vi "Set Photon Counting Threshold.vi"(8 "error in (no error)":errorcluster, 10 "max":i32, 11 "min":i32) -> (0 "error out":errorcluster, 3 "function return":u32)   [LabVIEW 2014, in "atmcd32d.lvlib"]
doc: "unsigned int WINAPI SetPhotonCountingThreshold(long min, long max);"
uses:
  atmcd32d.lvlib
  atmcd32d.dll
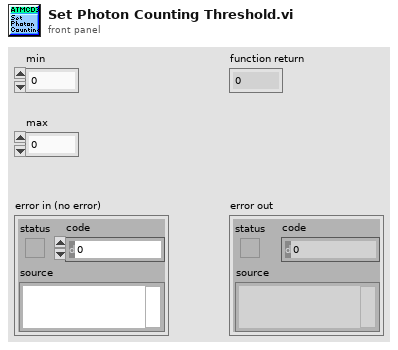
[diagram p1: front panel]
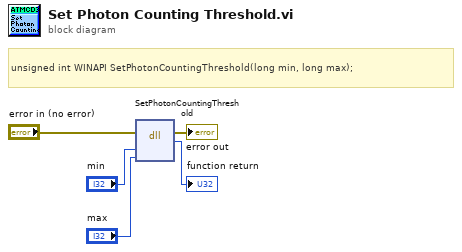
[diagram p0: block diagram]
diagram:
  # "unsigned int WINAPI SetPhotonCountingThreshold(long min, long max);"
  n1 = dll-call lib="C:/Users/Bakir/Documents/Lambda2-Testing/lib/Andorlib/atmcd32d.*" fn="SetPhotonCountingThreshold"(error in="error in (no error)", "min"="min", "max"="max") -> (error out=→"error out":errorcluster, →"function return":u32)  [unwired: 4 in, 1 out]
